vi "Set X Voltage.vi"(2 "X position (V)":dbl) -> ()   [LabVIEW 2014]
uses:
  global_channels.vi
  global_variables_AWG.vi
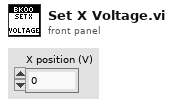
[diagram p1: front panel]
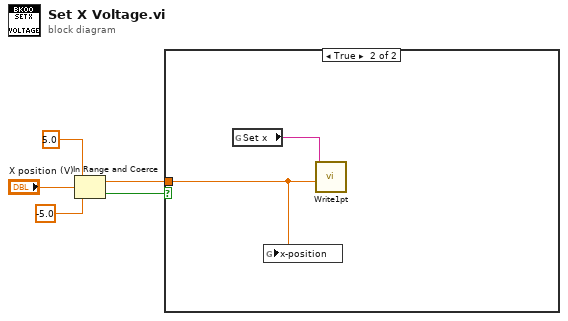
[diagram p0: block diagram]
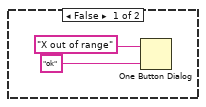
[diagram p2: hidden frame]
diagram:
  n1 = In Range and Coerce(upper limit=5.0, x="X position (V)", lower limit=-5.0) -> (coerced(x)=w1:dbl, In Range?=w2:bool)
  n2 = case shown="True" w2 {
    tunnel: w1 -> [_ w8]
    frame False {
      n3 = One Button Dialog(message="X out of range", button name ("OK")="ok") -> ()  [unwired: 1 out]
    }
    frame True {
      n4 = global read "global_channels.vi" "Set x"() -> (w9:tag)
      n5 = global write "global_variables_AWG.vi" "x-position"(w8) -> ()
      n6 = call "Write1pt.vi"("data"=w8, "physical channel"=w9) -> ()  [unwired: 10 in]
    }
  }
